vi "Read Screw Motor Config.vi"(8 "error in (no error)":errorcluster, 10 "Configuration In":variant, 11 "Climber in":refnum<class "Climber.lvclass">) -> (0 "error out":errorcluster, 3 "Climber out":refnum<class "Climber.lvclass">)   [LabVIEW 2019, in "Climber.lvlib" / "Climber.lvclass"]
uses:
  Climber.lvclass
  Controls/Screw Motor.ctl
  Climber.lvclass/Climber.ctl
  38ab3675-3df8-4b57-acd6-b773113a0650.vi
  7a57fc81-05ef-4779-90f3-325c55a1fd32.vi
  <vilib>/Utility/error.llb/Trim Whitespace.vi
  <vilib>/Utility/error.llb/Error Cluster From Error Code.vi
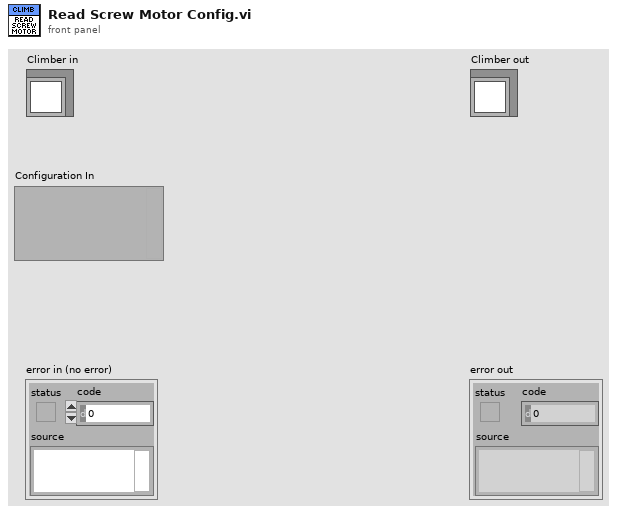
[diagram p1: front panel]
types:
  T1 = typedef "Climber.lvlib/Climber.lvclass/Screw Motor.ctl" = cluster{"Refnum Name":string, "CAN ID":u32, "I":dbl, "D":dbl, "P":dbl, "F":dbl, "Velocity":dbl, "Acceleration":dbl}
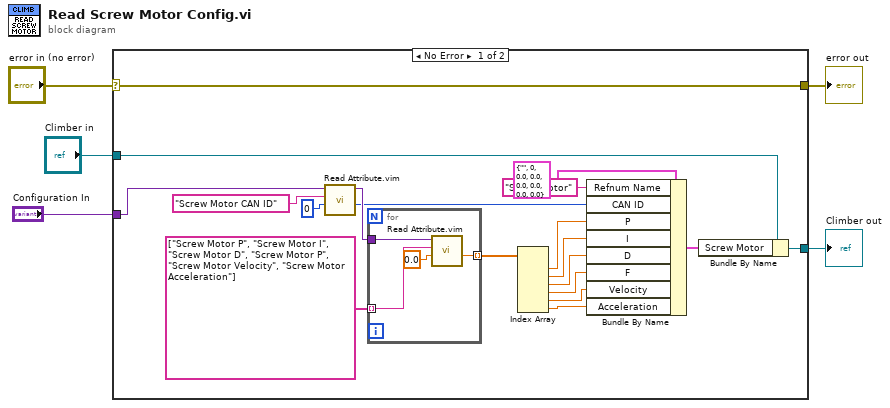
[diagram p0: block diagram]
diagram:
  n1 = case shown="No Error" "error in (no error)" {
    selector: "error in (no error)" -> [w20 w30]
    tunnel: [w20 w30] -> w4
    tunnel: [w7 w29] -> w2
    tunnel: "Climber in" -> [w9 w29]
    tunnel: "Configuration In" -> [w23 _]
    frame No Error {
      n2 = call "Read Attribute.vim"("default value (data type)"=u32 0, "name"="Screw Motor CAN ID", "variant in"=w23) -> ("value"=w18:u32, "variant out"=w21:variant)  [unwired: 5 in, 2 out]
      n3 = for {
        tunnel: string[] ["Screw Motor P", "Screw Motor I", "Screw Motor D", "Screw Motor P", "Screw Motor Velocity", "Screw Motor Acceleration"] -> [w28] mode=indexing
        tunnel: w21 -> [w27]
        tunnel: [w25] -> w17 mode=indexing
        n4 = call "Read Attribute.vim"("default value (data type)"=0.0, "name"=w28, "variant in"=w27) -> ("value"=w25:dbl)  [unwired: 5 in, 3 out]
      }
      n5 = Index Array(array=w17) -> (element #1=w16:dbl, element #2=w15:dbl, element #3=w14:dbl, element #4=w13:dbl, element #5=w12:dbl, element #6=w11:dbl)  [unwired: 6 in]
      n6 = Bundle By Name(cluster=T1 {"Refnum Name"="", "CAN ID"=0, "I"=0.0, "D"=0.0, "P"=0.0, "F"=0.0, "Velocity"=0.0, "Acceleration"=0.0} ("Screw Motor"), "Refnum Name"="Screw Motor", "CAN ID"=w18, "P"=w16, "I"=w15, "D"=w14, "F"=w13, "Velocity"=w12, "Acceleration"=w11) -> (w8:T1)
      n7 = Bundle By Name(cluster=w9, "Screw Motor"=w8) -> (w7:refnum<class "Climber.lvclass">)
    }
    frame Error {
    }
  }
  "error out" <- w4
  "Climber out" <- w2
